vi "Sequences Initialization Test.vi"() -> (0 "error out":errorcluster, 2 "Pass":bool)   [LabVIEW 2015, in "Sequencer Module tests.lvlib"]
uses:
  Sequencer Module tests.lvlib
  classes/Sequence/Execution/Sequence.lvclass
  classes/Sequence/Config/Sequence Config.lvclass
  <vilib>/NI/Tag Bus Module Framework/channel/TBM channel.lvclass
panel:
  out "Names":string[](array[string])
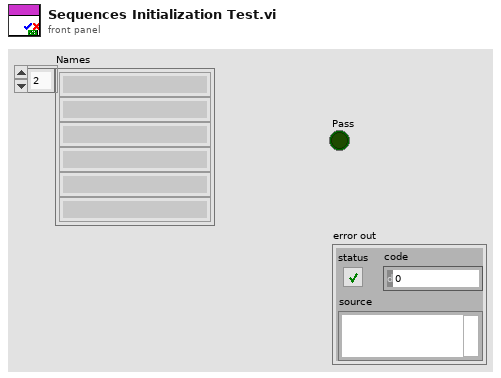
[diagram p1: front panel]
types:
  T1 = typedef "Sequencer Module configuration.lvclass/Line.ctl" = cluster{"Sequence":refnum<class "Sequence Config.lvclass">}
  T2 = typedef "TBM channel.lvclass/data tables.ctl" = cluster{"input data":T3, "processing parameter":T3, "processing result":T3, "output data":T3}
  T3 = typedef "tag bus.lvlib/dictionary table pair.ctl" = cluster{"data dictionary":refnum<class "data dictionary.lvclass">, "data table":T4}
  T4 = typedef "tag bus.lvlib/data table.lvlib/data table.ctl" = cluster{"Double":dbl[], "Single":sgl[], "I64":i64[], "I32":i32[], "I16":i16[], "I8":i8[], "U64":u64[], "U32":u32[], "U16":u16[], "U8":u8[], "Boolean":bool[], "String":string[], "Array of Double":cluster{"DBL Array":dbl[]}[], "Array of Single":cluster{"SGL Array":sgl[]}[], "Array of I64":cluster{"I64 Array":i64[]}[], "Array of I32":cluster{"I32 Array":i32[]}[], "Array of I16":cluster{"I16 Array":i16[]}[], "Array of I8":cluster{"I8 Array":i8[]}[], "Array of U64":cluster{"U64 Array":u64[]}[], "Array of U32":cluster{"U32 Array":u32[]}[], "Array of U16":cluster{"U16 Array":u16[]}[], "Array of U8":cluster{"U8 Array":u8[]}[], "Array of Boolean":cluster{"Boolean Array":bool[]}[], "Array of String":cluster{"String Array":string[]}[]}
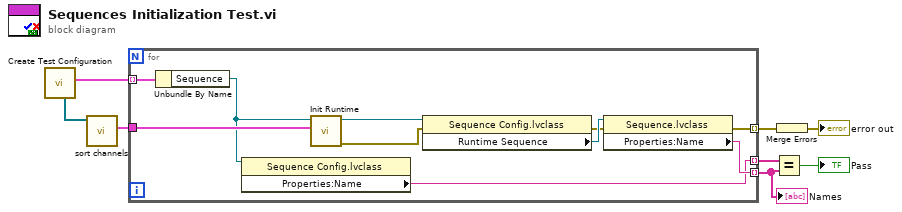
[diagram p0: block diagram]
diagram:
  n1 = call "Create Test Configuration.vi"() -> ("Lines"=w8:T1[], "Channels"=w7:refnum<class "TBM channel.lvclass">[])  [unwired: 6 in, 4 out]
  n2 = call <vilib>:"sort channels.vi"("channels in"=w7) -> ("data allocations"=w6:T2)  [unwired: 8 in, 2 out]
  n3 = for {
    tunnel: w8 -> [w15] mode=indexing
    tunnel: w6 -> [w16]
    tunnel: [w12] -> w5 mode=indexing
    tunnel: [w11] -> w2 mode=indexing
    tunnel: [w9] -> w3 mode=indexing
    n4 = Unbundle By Name(w15) -> ("Sequence"=w10:refnum<class "Sequence Config.lvclass">)
    n5 = property class="Sequence Config.lvclass"(reference=w10) -> ("Properties:Name"=w9:string)  [unwired: 1 in, 2 out]
    n6 = call-dynamic "Init Runtime.vi"("data allocations"=w16, "Sequence Config in"=w10) -> ("error out"=w14:errorcluster, "Sequence Config out"=w17:refnum<class "Sequence Config.lvclass">)  [unwired: 8 in]
    n7 = property class="Sequence Config.lvclass"(reference=w17, error in=w14) -> (error out=w13:errorcluster, "Runtime Sequence"=w18:refnum<class "Sequence.lvclass">)  [unwired: 1 out]
    n8 = property class="Sequence.lvclass"(reference=w18, error in=w13) -> (error out=w12:errorcluster, "Properties:Name"=w11:string)  [unwired: 1 out]
  }
  "Names" <- w2
  n9 = Equal?(x=w3, y=w2) -> (x = y?=→"Pass":bool)
  n10 = Merge Errors(w5) -> (→"error out":errorcluster)
